vi "Update Fan Status.vi"(8 "error in (no error)":errorcluster, 9 "Fan B":cluster{"State":bool, "Fault":bool}, 10 "Fan A":cluster{"State":bool, "Fault":bool}, 11 "Cooler in":refnum<class "Cooler.lvclass">) -> (0 "error out":errorcluster, 3 "Cooler out":refnum<class "Cooler.lvclass">)   [LabVIEW 2012, in "Cooler.lvlib" / "Cooler.lvclass"]
uses:
  Cooler.lvclass
  Cooler.lvclass/Cooler.ctl
  Cooler UI/Cooler UI with Events Messages/Update Fan Msg/Update Fan Msg.lvclass/Update Fan Msg.ctl
  <vilib>/ActorFramework/Message Enqueuer/Message Enqueuer.lvclass/Message Enqueuer.ctl
  <vilib>/ActorFramework/Message Enqueuer/Enqueue.vi
  <vilib>/ActorFramework/Message Priority Queue/Priority Enqueue.vi
  Cooler UI/Cooler UI with Events Messages/Update Fan Msg/Update Fan Msg.lvclass
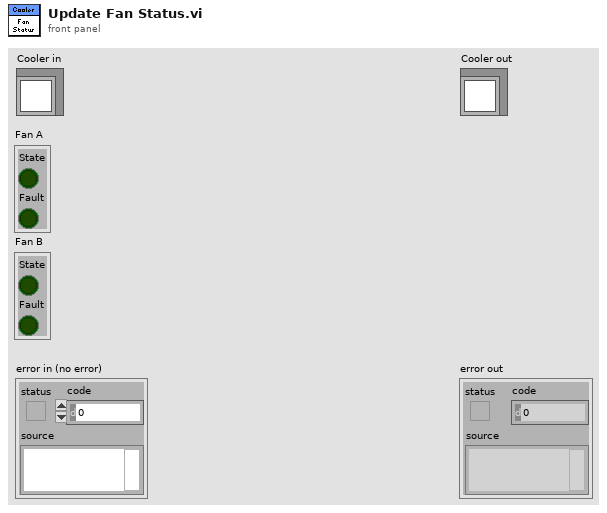
[diagram p1: front panel]
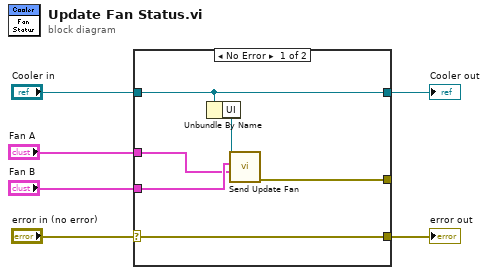
[diagram p0: block diagram]
diagram:
  n1 = case shown="No Error" "error in (no error)" {
    selector: "error in (no error)" -> [w12 w14]
    tunnel: [w12 w14] -> w5
    tunnel: [w9 w13] -> w3
    tunnel: "Cooler in" -> [w9 w13]
    tunnel: "Fan A" -> [w10 _]
    tunnel: "Fan B" -> [w11 _]
    tunnel: [w7 _] -> _
    frame No Error {
      n2 = Unbundle By Name(w9) -> ("UI"=w8:refnum<class "Message Enqueuer.lvclass">)
      n3 = call "Send Update Fan.vi"("Fan A"=w10, "Fan B"=w11, "Message Enqueuer"=w8) -> ("error out"=w7:errorcluster)  [unwired: 7 in, 1 out]
    }
    frame Error {
    }
  }
  "error out" <- w5
  "Cooler out" <- w3
